vi "选择测试环节.vi"(1 "当前状态":T2=enum."提示消息", 2 "测试选项":T1={"指令测试"=TRUE, "特殊功能测试"=TRUE, "数据测试"=TRUE, "心跳包测试"=TRUE, "升级测试"=TRUE, "中心切换测试"=TRUE, "生成报告"=TRUE}) -> (0 "下一步状态":T2=enum."提示消息")   [LabVIEW 2015]
panel:
  out "数组":bool[](array[boolean])
  out "布尔文本.文本":string
  out "数字显示.文本":string
  out "字符串[]":string[](array[string])
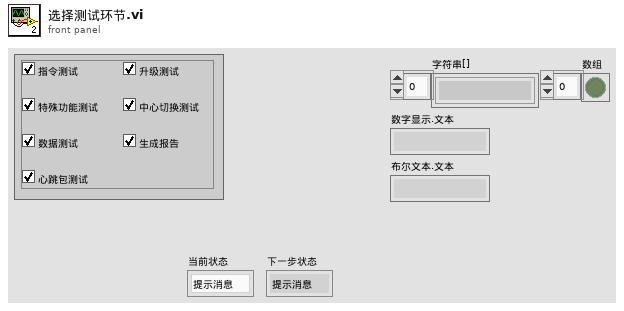
[diagram p1: front panel]
types:
  T1 = typedef "测试项目.ctl" = cluster{"指令测试":bool, "特殊功能测试":bool, "数据测试":bool, "心跳包测试":bool, "升级测试":bool, "中心切换测试":bool, "生成报告":bool}
  T2 = typedef "状态机状态.ctl" = enum16{"初始化", "等待按键", "串口操作", "检索模块", "网络测试", "测试项目", "指令测试", "数据测试", "特殊功能测试", "心跳包测试", "升级测试", "中心切换", "生成报表", "提示消息", "退出"}
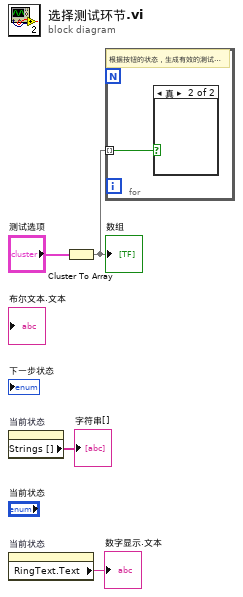
[diagram p0: block diagram]
diagram:
  n1 = property on="当前状态" class="Enum (严格)"() -> ("Strings []"=→"字符串[]":string[])  [unwired: 2 in, 2 out]
  n2 = property on="当前状态" class="Enum (严格)"() -> ("RingText.Text"=→"数字显示.文本":string)  [unwired: 2 in, 2 out]
  n3 = Cluster To Array(cluster="测试选项") -> (array=w1:bool[])
  "数组" <- w1
  n4 = for {
    tunnel: w1 -> [w5] mode=indexing
    # "根据按钮的状态，生成有效的测试数组"
    n5 = case shown="真" w5 {
      frame False {
      }
      frame True {
      }
    }
  }
